vi "readFromXML.vi"(8 "error in (no error)":errorcluster, 10 "XMLin":string, 11 "ScienceTargetConfiguration in":refnum<class "ScienceTargetConfiguration.lvclass">) -> (0 "error out":errorcluster, 3 "ScienceTargetConfiguration out":refnum<class "ScienceTargetConfiguration.lvclass">)   [LabVIEW 2014, in "TCSDataDefinitions.lvlib" / "TCSCommand.lvlib" / "TargetConfiguration.lvlib" / "ScienceTargetConfiguration.lvclass"]
uses:
  ScienceTargetConfiguration.lvclass
  ScienceTargetConfiguration.lvclass/ScienceTargetConfiguration.ctl
  TargetConfiguration/TargetConfiguration.lvclass
  Rotator/Rotator.lvclass
  <userlib>/Common/XML/XMLParser/XMLParser.lvclass
panel:
  out "fracrate":dbl
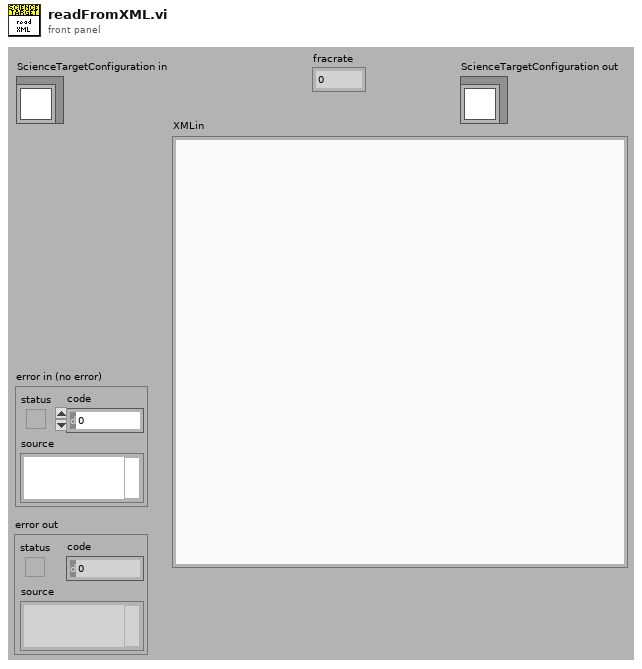
[diagram p1: front panel]
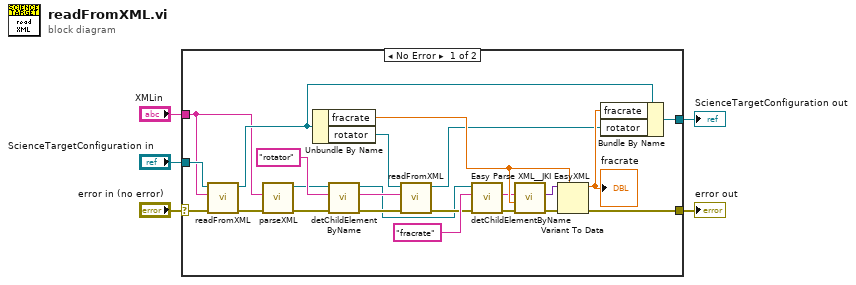
[diagram p0: block diagram]
diagram:
  n1 = case shown="No Error" "error in (no error)" {
    selector: "error in (no error)" -> [w21 w30]
    tunnel: [w12 w30] -> w4
    tunnel: [w20 w29] -> w2
    tunnel: "ScienceTargetConfiguration in" -> [w28 w29]
    tunnel: "XMLin" -> [w25 _]
    frame No Error {
      n2 = call-parent "readFromXML.vi"("error in (no error)"=w21, "XMLin"=w25, "TargetConfiguration in"=w28) -> ("error out"=w26:errorcluster, "TargetConfiguration out"=w27:refnum<class "ScienceTargetConfiguration.lvclass">)  [unwired: 7 in]
      n3 = call <userlib>:"parseXML.vi"("error in (no error)"=w26, "XMLString in"=w25) -> ("error out"=w23:errorcluster, "Element out"=w7:refnum<class "XMLParser.lvclass">)  [unwired: 8 in]
      n4 = Unbundle By Name(w27) -> ("fracrate"=w11:dbl, "rotator"=w17:refnum<class "Rotator.lvclass">)
      n5 = call <userlib>:"detChildElementByName.vi"("error in (no error)"=w23, "childName"="rotator" ("ChildName"), "Element in"=w7) -> ("error out"=w15:errorcluster, "childXML"=w16:string, "Element out"=w6:refnum<class "XMLParser.lvclass">)  [unwired: 5 in, 1 out]
      n6 = call-dynamic "readFromXML.vi"("error in (no error)"=w15, "XML in"=w16, "Rotator in"=w17) -> ("error out"=w14:errorcluster, "Rotator out"=w9:refnum<class "Rotator.lvclass">)  [unwired: 7 in]
      n7 = call <userlib>:"detChildElementByName.vi"("error in (no error)"=w14, "childName"="fracrate" ("ChildName"), "Element in"=w6) -> ("error out"=w13:errorcluster, "childXML"=w8:string)  [unwired: 5 in, 2 out]
      n8 = call <vilib>:"Easy Parse XML__JKI EasyXML.vi"("error in (no error)"=w13, "LabVIEW Data (Type)"=w11, "XML String"=w8) -> ("error out"=w19:errorcluster, "LabVIEW Data"=w18:variant)  [unwired: 7 in]
      n9 = Variant To Data(error in=w19, type=w11, Variant=w18) -> (data=w10:dbl, error out=w12:errorcluster)
      "fracrate" <- w10
      n10 = Bundle By Name(cluster=w27, "fracrate"=w10, "rotator"=w9) -> (w20:refnum<class "ScienceTargetConfiguration.lvclass">)
    }
    frame Error {
    }
  }
  "error out" <- w4
  "ScienceTargetConfiguration out" <- w2
